vi "Read Instrument Data.vi"(8 "error in (no error)":errorcluster {"code" format="%.0x"}, 10 "number of bytes to read (0)":i32, 11 "VISA Resource Name":refnum<visa-resource-name>) -> (0 "error out":errorcluster {"code" format="%.0x"}, 1 "num bytes read":i32, 2 "read buffer":string, 3 "VISA Resource Name Out":refnum<visa-resource-name>)   [LabVIEW 2011, in "Agilent 546XX Series.lvlib"]
doc: "This VI reads data from the instrument."
uses:
  Agilent 546XX Series.lvlib
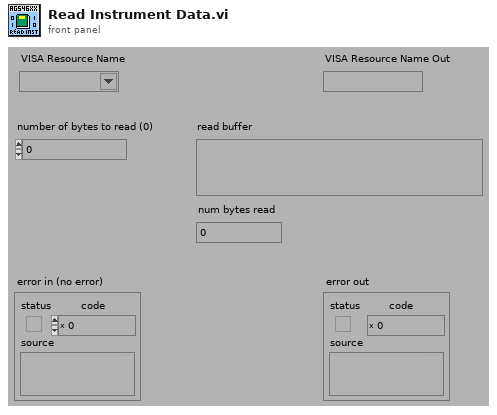
[diagram p1: front panel]
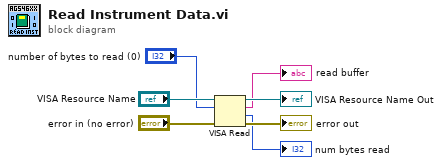
[diagram p0: block diagram]
diagram:
  n1 = VISA Read(VISA resource name="VISA Resource Name", byte count="number of bytes to read (0)", error in (no error)="error in (no error)") -> (VISA resource name out=→"VISA Resource Name Out":refnum<visa-resource-name>, read buffer=→"read buffer":string, return count=→"num bytes read":u32, error out=→"error out":errorcluster)
